vi "int32 to Hex.vi"(11 "number":dbl) -> (3 "Hex string":string)   [LabVIEW 2017]
panel:
  out "concatenated string":string
  # "RE-ENTRANT"
  # "SUBROUTINE"
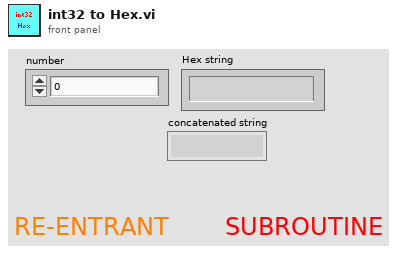
[diagram p1: front panel]
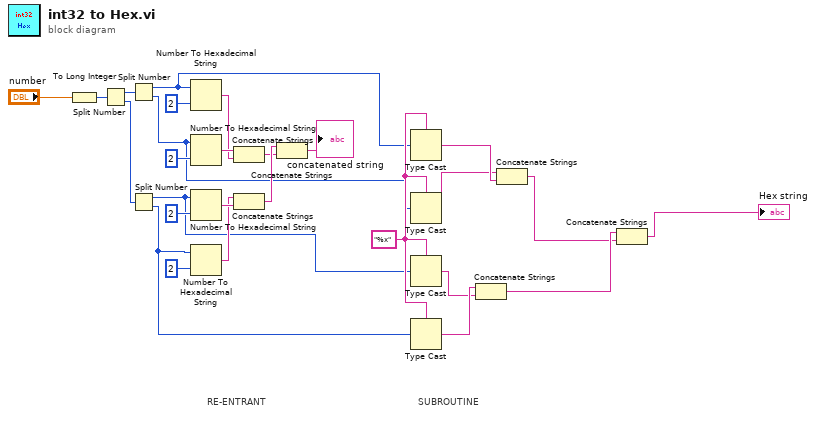
[diagram p0: block diagram]
diagram:
  w13 = "%x" ("type")
  # "SUBROUTINE"
  # "RE-ENTRANT"
  n1 = To Long Integer(number="number") -> (32bit integer=w20:i32)
  n2 = Split Number(x=w20) -> (hi(x)=w26:u16, lo(x)=w27:u16)
  n3 = Split Number(x=w26) -> (hi(x)=w10:u8, lo(x)=w11:u8)
  n4 = Split Number(x=w27) -> (hi(x)=w12:u8, lo(x)=w3:u8)
  n5 = Number To Hexadecimal String(1:i16 2 ("width (-)"), 2:w10) -> (0:w14:string)
  n6 = Number To Hexadecimal String(1:i16 2 ("width (-)"), 2:w11) -> (0:w23:string)
  n7 = Number To Hexadecimal String(1:i16 2 ("width (-)"), 2:w12) -> (0:w25:string)
  n8 = Number To Hexadecimal String(1:i16 2 ("width (-)"), 2:w3) -> (0:w24:string)
  n9 = Concatenate Strings(w23, w14) -> (w21:string)
  n10 = Concatenate Strings(w24, w25) -> (w22:string)
  n11 = Concatenate Strings(w22, w21) -> (→"concatenated string":string)
  n12 = Type Cast(type=w13, x=w10) -> (*(type *) &x=w7:string)
  n13 = Type Cast(type=w13, x=w11) -> (*(type *) &x=w6:string)
  n14 = Type Cast(type=w13, x=w12) -> (*(type *) &x=w8:string)
  n15 = Type Cast(type=w13, x=w3) -> (*(type *) &x=w9:string)
  n16 = Concatenate Strings(w9, w8) -> (w5:string)
  n17 = Concatenate Strings(w6, w7) -> (w4:string)
  n18 = Concatenate Strings(w5, w4) -> (→"Hex string":string)
